vi "Dashboard Main.vi"() -> ()   [LabVIEW 2013]
uses:
  <vilib>/event_ctls.llb/eventvkey.ctl
  <vilib>/Rock Robotics/WPI/Dashboard/WPI_DashboardLogging Global.vi
  <vilib>/Utility/config.llb/Write Key (String).vi
  <vilib>/Utility/config.llb/Write Key (I32).vi
  <vilib>/Utility/config.llb/NI_LVConfig.lvlib
panel:
  out "Image Message":string="Timeout in Camera Communications"
  in  "Rec Mode":enum32{"Stop", "Record", "Playback"}(radio)
  in  "Dashboard Tab":T1(tab)
  in  "DriverValue":string(combo)
  in  "Camera Settings":T2={"Frame Rate"=30, "Compression"=30, "Size"=1} {"Frame Rate" scale=1.0..30.0; "Size" items=["640x480", "320x240", "160x120"]}
  out "MotorSliders R":cluster{"MotorSlide1":dbl, "MotorSlide2":dbl} {"MotorSlide2" scale=-1.0..1.0 scale format="%#_2e"; "MotorSlide1" scale=-1.0..1.0 scale format="%#_2e"}
  out "MotorChart R":cluster{"Numeric":dbl, "Numeric":dbl}(graph)
  out "MotorSliders L":T3 {"MotorSlide4 2" scale=0.0..14.0 scale format="%#_2e"; "MotorSlide2" scale=-1.0..1.0 scale format="%#_2e"; "MotorSlide1" scale=-1.0..1.0 scale format="%#_2e"}
  out "MotorChart L":T4(graph)
  out "JS1 Z":dbl(slide) scale=-1.0..1.0 scale format="%#_2e"
  out "Joystick 1":cluster{"X":dbl, "Y":dbl}[](graph)
  out "JS Buttons 1":T5
  out "JS2 Z":dbl(slide) scale=-1.0..1.0 scale format="%#_2e"
  out "Joystick 2":cluster{"X":dbl, "Y":dbl}[](graph)
  out "JS Buttons 2":T5
  out "Mode":T6(ring)=enum."Auto Disabled"
  out "Camera IP":string
  in  "DB Camera Config":bool
  out "fps":dbl format="%#.1g"
  out "Mbps":dbl format="%#.1g"
  out "Mbps 2":bool
  out "LED 1":bool
  in  "Slider 1":dbl(slide) scale=0.0..100.0
  in  "Checkbox 2":bool
  in  "Checkbox 1":bool
  in  "Test Slider":dbl(slide) scale=0.0..100.0 scale format="%#_3g"
  in  "On/Off":bool caption="Solenoid"
  in  "Test Name":u16(ring) items=["Select the test to run...", "Example Test", "-------------------------------", "List of tests is built in robot code.", "Replace with your own automated tests."]
  in  "Test Tree":string(tree)
  in  "Motor":cluster{"Value":dbl, "Enable":bool} {"Value" scale=-1.0..1.0 scale format="%#_3g"}
  out "Progress":T7 {"Test Progress" scale=0.0..100.0}
  in  "Rev/Fwd":cluster{"Forward":bool, "Reverse":bool}
  in  "Test Ring":u16(ring) items=["Auto", "Fixed indoor", "Fixed outdoor 1", "Fixed outdoor 2", "Fixed fluorescent 1", "Fixed fluorescent 2", "Hold current"]
  in  "Listbox":i32(listbox)
  out "Tree":string(tree)
  out "Camera Image":T8(plugin-control)
  in  "Enable":bool
  # "Left"
  # "Front"
  # "Right"
  # "Battery"
  # "Customize by placing controls and indicators here and name to\nmatch Dashboard Variables on robot."
  # "This tab is a great place for autonomous settings and validation.\nCustomize by placing controls and indicators here and name to\nmatch Dashboard Variables on robot."
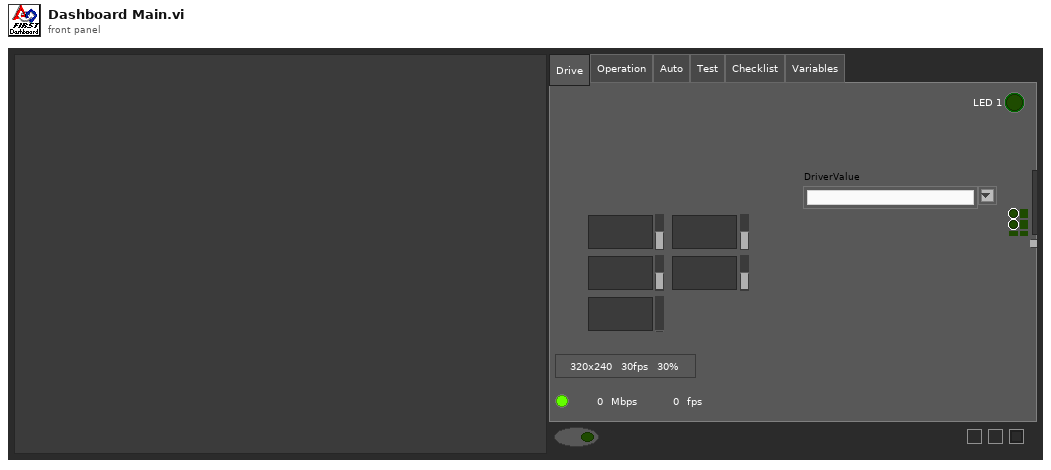
[diagram p1: front panel]
types:
  T1 = enum32{"Drive", "Operation", "Auto", "Test", "Checklist", "Variables"}
  T2 = cluster{"Frame Rate":i32, "Compression":i32, "Size":u16}
  T3 = cluster{"MotorSlide1":dbl, "MotorSlide2":dbl, "MotorSlide4 2":dbl}
  T4 = cluster{"Numeric":dbl, "Numeric":dbl, "Battery":sgl}
  T5 = cluster{bool, bool, bool, bool, bool, bool, bool, bool, bool, bool, bool, bool}
  T6 = enum8{"Tele-Op Disabled", "Tele-Op Enabled", "Auto Disabled", "Auto Enabled", "Test Disabled", "Test Enabled", ""}
  T7 = cluster{"Test Progress":u8, "Test Progress Text":string}
  T8 = typedef "IMAQ Image.ctl" = refnum<image>
  T9 = typedef "Image Type" = u32
  T10 = cluster{"Digital Inputs":bool[], "Digital Outputs":bool[]}
  T11 = cluster{"Competition mode":bool, "Robot Link":bool, "Autonomous":bool, "Enabled":bool, "E-Stop":bool, "Simulated":bool, "TestMode":bool, "Docked Window":bool}
  T12 = cluster{"Boolean Array[0]":bool, "Boolean Array[1]":bool, "Boolean Array[2]":bool, "Boolean Array[3]":bool, "Boolean Array[4]":bool, "Boolean Array[5]":bool, "Boolean Array[6]":bool, "Boolean Array[7]":bool, "Boolean Array[8]":bool, "Boolean Array[9]":bool, "Boolean Array[10]":bool, "Boolean Array[11]":bool}
  T13 = typedef "NI_LVConfig.lvlib/Config Data RefNum.ctl" = refnum<k1>
  T14 = typedef "eventvkey.ctl" = enum16{"ASCII", "Enter", "Return", "Shift", "Ctrl", "Alt", "Cmd", "Opt", "Caps", "NumLock", "Clear", "Break", "Up", "Down", "Left", "Right", "Insert", "Delete", "Home", "End", "PageUp", "PageDown", "Escape", "Help", "Pause", "ScrollLock", "F1", "F2", "F3", "F4", "F5", "F6", "F7", "F8", "F9", "F10", "F11", "F12", "F13", "F14", "F15", "F16", "F17", "F18", "F19", "F20", "F21", "F22", "F23", "F24", "Play", "VolumeUp", "VolumeDown", "Mute", "Two Byte Char"}
  T15 = cluster{"Image Size":bool, "Image Type":bool, "Pixel Value":bool, "ROI Information":bool, "Zoom Factor":bool}
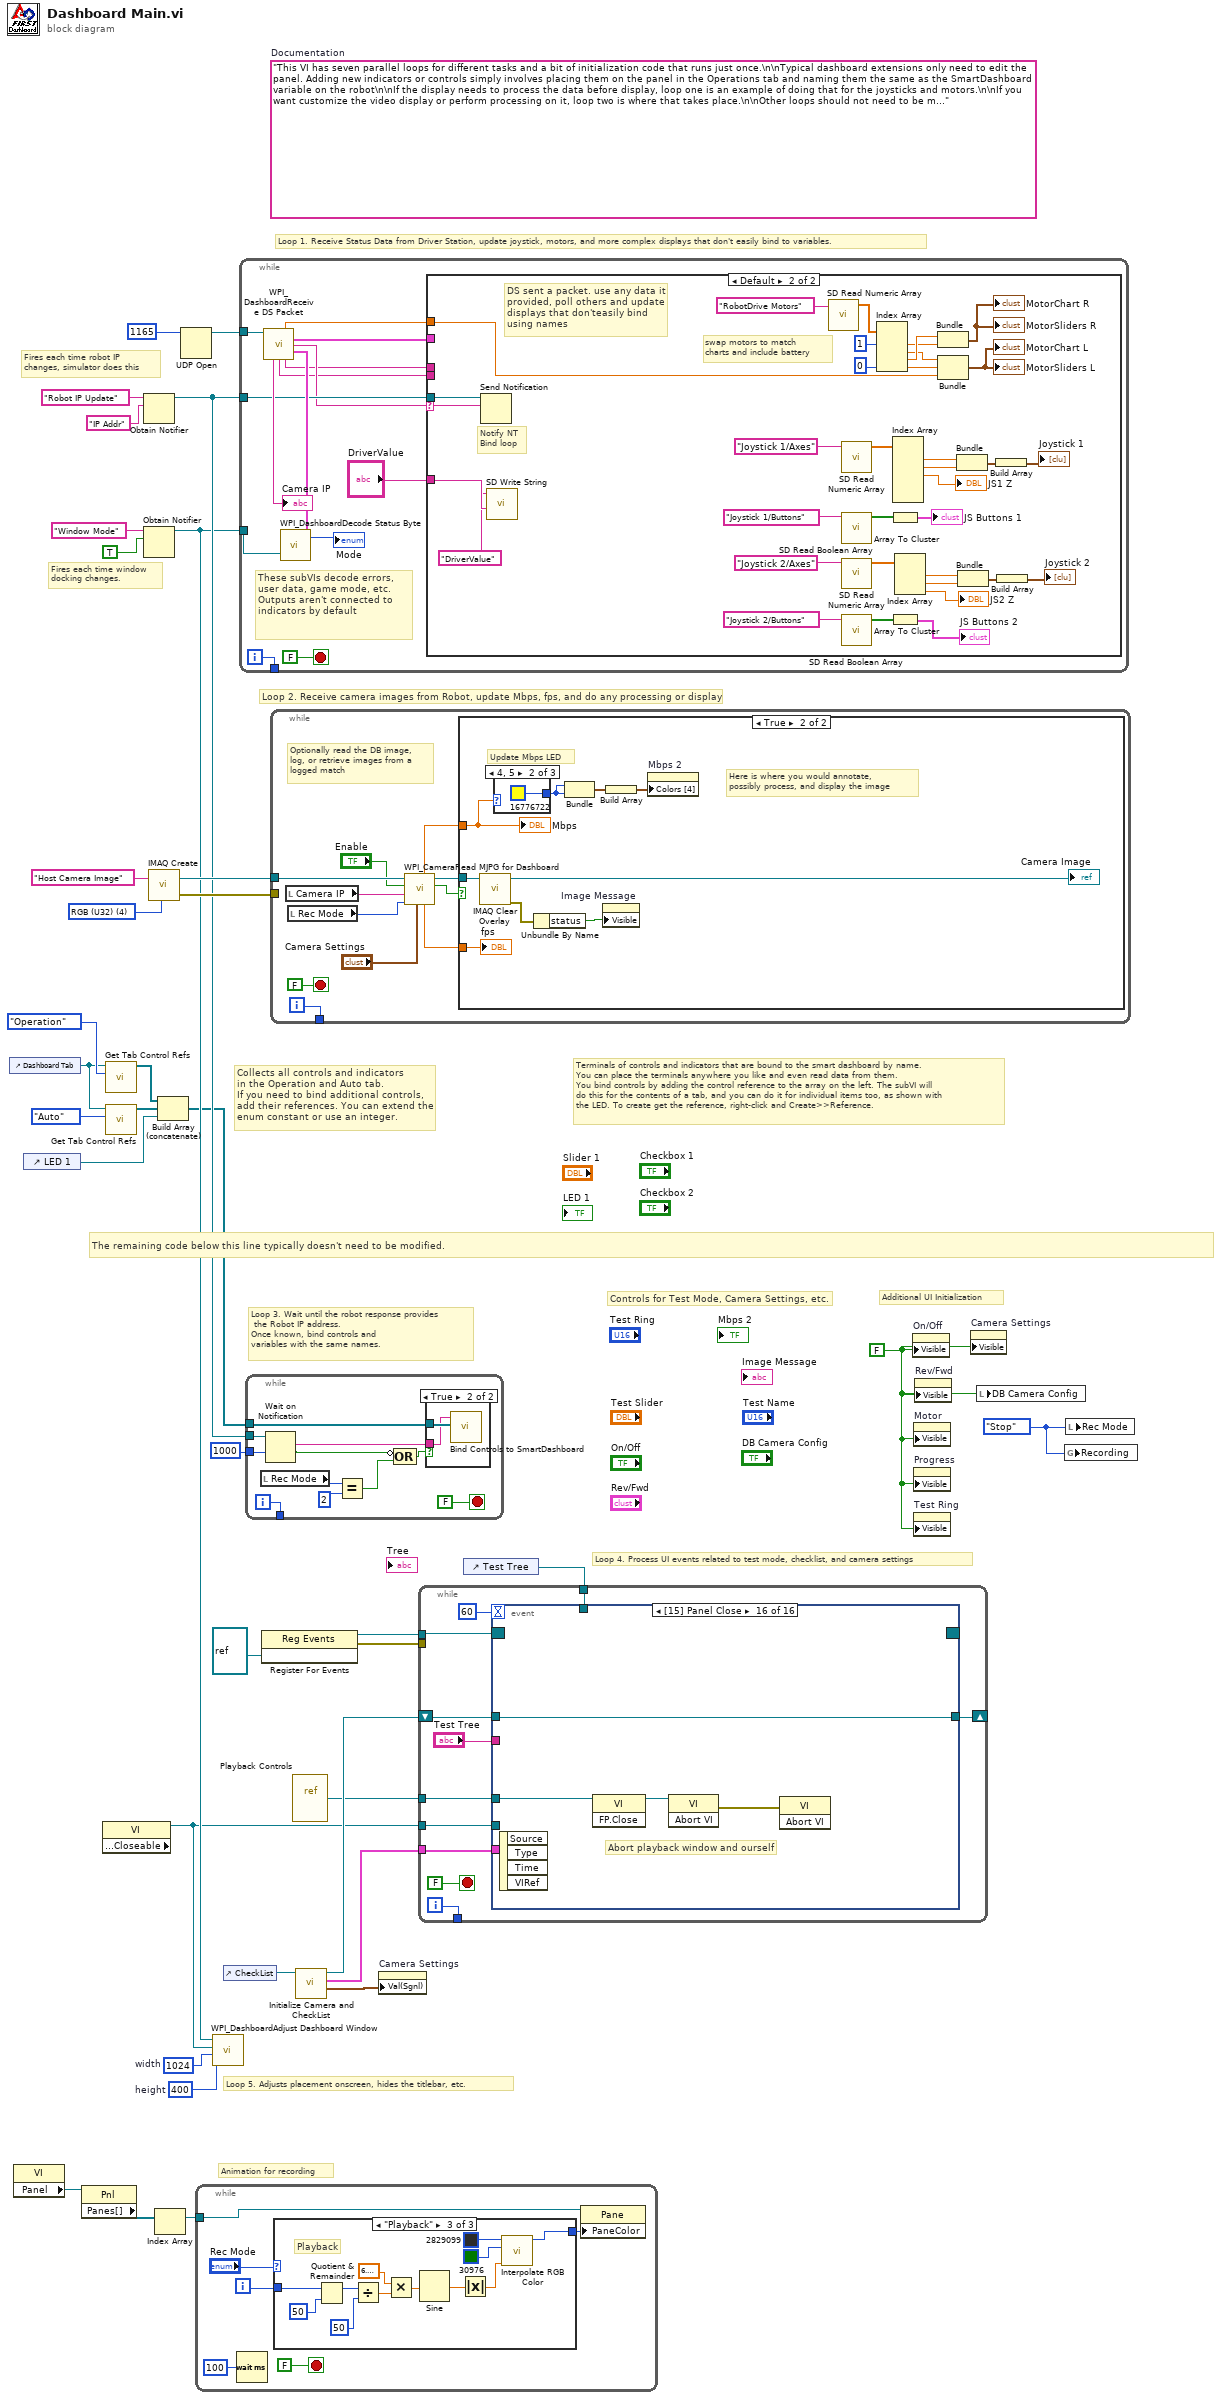
[diagram p0: block diagram]
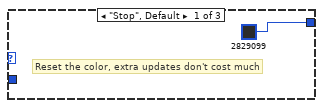
[diagram p2: hidden frame]
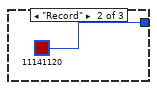
[diagram p3: hidden frame]
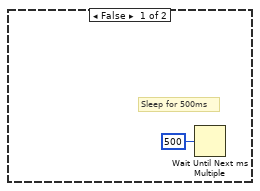
[diagram p5: hidden frame]
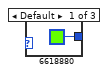
[diagram p6: hidden frame]
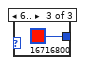
[diagram p7: hidden frame]
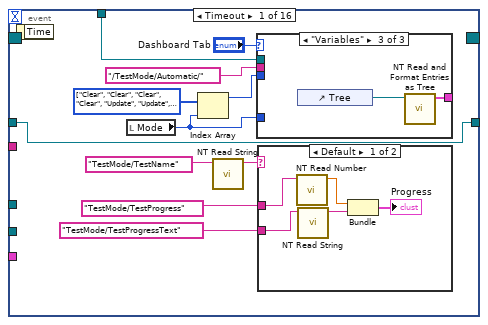
[diagram p8: hidden frame]
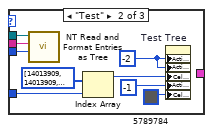
[diagram p10: hidden frame]
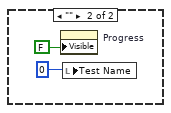
[diagram p11: hidden frame]
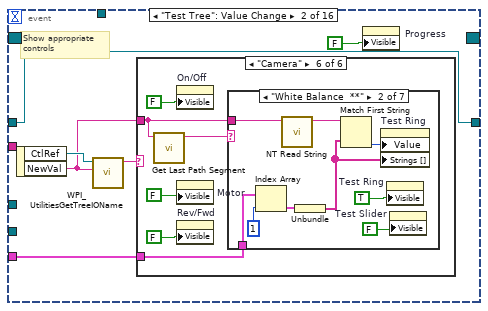
[diagram p12: hidden frame]
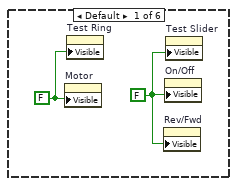
[diagram p13: hidden frame]
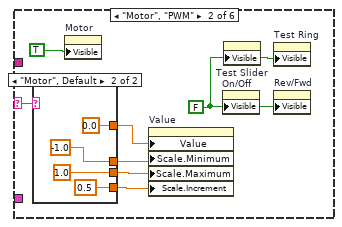
[diagram p14: hidden frame]
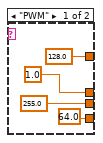
[diagram p15: hidden frame]
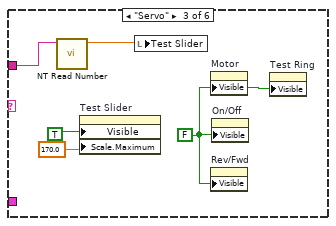
[diagram p16: hidden frame]
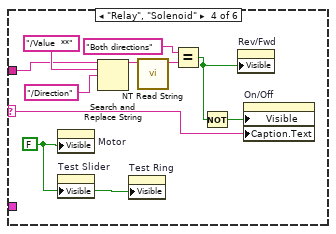
[diagram p17: hidden frame]
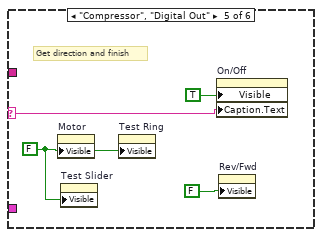
[diagram p18: hidden frame]
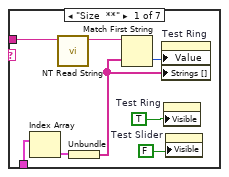
[diagram p19: hidden frame]
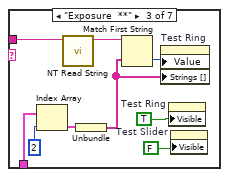
[diagram p20: hidden frame]
diagram:
  w8 = enum32{"Stop", "Record", "Playback"}."Stop" ("Rec Mode")
  w11 = 400  # height
  w12 = 1024  # width
  w25 = FALSE ("Visible")
  (unwired) "This VI has seven parallel loops for different tasks and a bit of initialization code that runs just once.\n\nTypical dashboard extensions only need to edit the panel. Adding new indicators or controls simply involves placing them on the panel in the Operations tab and naming them the same as the SmartDashboard variable on the robot\n\nIf the display needs to process the data before display, loop one is an example of doing that for the joysticks and motors.\n\nIf you want customize the video display or perform processing on it, loop two is where that takes place.\n\nOther loops should not need to be modified. They are pretty standard, and document the task they perform."  # Documentation
  w35 = T9 4 items=["Grayscale (U8)", "Grayscale (I16)", "Grayscale (SGL)", "Complex (CSG)", "RGB (U32)", "HSL (U32)", "RGB (U64)"] ("Image Type")
  # "Controls for Test Mode, Camera Settings, etc."
  # "Additional UI Initialization"
  # "Animation for recording"
  # "Fires each time robot IP\nchanges, simulator does this"
  # "Fires each time window\ndocking changes."
  # "Collects all controls and indicators\nin the Operation and Auto tab.\nIf you need to bind additional controls,\nadd their references. You can extend the\nenum constant or use an integer."
  # "The remaining code below this line typically doesn't need to be modified."
  # "Loop 4. Process UI events related to test mode, checklist, and camera settings"
  # "Terminals of controls and indicators that are bound to the smart dashboard by name.\nYou can place the terminals anywhere you like and even read data from them.\nYou bind controls by adding the control reference to the array on the left. The subVI will\ndo this for the contents of a tab, and you can do it for individual items too, as shown with\nthe LED. To create get the reference, right-click and Create>>Reference."
  # "Loop 3. Wait until the robot response provides\n the Robot IP address.\nOnce known, bind controls and\nvariables with the same names."
  # "Loop 5. Adjusts placement onscreen, hides the titlebar, etc."
  # "Loop 1. Receive Status Data from Driver Station, update joystick, motors, and more complex displays that don't easily bind to variables."
  # "Loop 2. Receive camera images from Robot, update Mbps, fps, and do any processing or display"
  n1 = control-ref of="Dashboard Tab"() -> (w6:refnum<vi>)
  n2 = property class="VI"() -> ("Panel"=w19:refnum<vi>)  [unwired: 2 in, 2 out]
  n3 = control-ref of="LED 1"() -> (w1:refnum<vi>)
  n4 = property class="Pnl"(reference=w19) -> ("Panes[]"=w20:refnum<vi>[])  [unwired: 1 in, 2 out]
  n5 = property class="VI" props=["Front Panel.Closeable"]() -> (reference out=w7:refnum<vi>)  [unwired: 2 in, 2 out]
  n6 = call <vilib>:"Get Tab Control Refs.vi"("Page Index"=T1."Operation" ("Dashboard Tab"), "TabControl in"=w6) -> ("ControlsOnPage"=w4:refnum<vi>[])  [unwired: 9 in]
  n7 = call <vilib>:"Get Tab Control Refs.vi"("Page Index"=T1."Auto" ("Dashboard Tab"), "TabControl in"=w6) -> ("ControlsOnPage"=w5:refnum<vi>[])  [unwired: 9 in]
  n8 = Obtain Notifier(name (unnamed)="Robot IP Update", notification data type="IP Addr" ("name (unnamed)")) -> (notifier out=w29:refnum<notifier>)  [unwired: 2 in, 2 out]
  n9 = Obtain Notifier(name (unnamed)="Window Mode", notification data type=TRUE) -> (notifier out=w10:refnum<notifier>)  [unwired: 2 in, 2 out]
  n10 = call "IMAQ Create"("Image Name"="Host Camera Image", "Image Type"=w35) -> ("New Image"=w33:T8, "error out"=w32:errorcluster)  [unwired: 2 in, 1 out]
  n11 = Index Array(array=w20) -> (element=w18:refnum<vi>)  [unwired: 1 in]
  n12 = Build Array (concatenate)(w4, w5, w1) -> (w3:refnum<vi>[])
  n13 = UDP Open(11:u16 1165 ("port")) -> (port=w36:refnum<k16>)  [unwired: 2 in, 4 out]
  n14 = while {
    tunnel: w18 -> [w39]
    i -> [w42]
    stop <- FALSE stop-if-true
    n15 = Wait (ms)(milliseconds to wait=u32 100) -> ()  [unwired: 1 out]
    n16 = case shown="\"Playback\"" "Rec Mode" {
      tunnel: w42 -> [_ _ w57]
      tunnel: [u32 2829099 ("Base Color") u32 11141120 ("Target Color") w46] -> w38
      frame "Stop", Default {
        # "Reset the color, extra updates don't cost much"
      }
      frame "Record" {
      }
      frame "Playback" {
        # "Playback"
        n17 = Quotient & Remainder(x=w57, y=u32 50 ("milliseconds to wait")) -> (x-y*floor(x/y)=w53:u32)  [unwired: 1 out]
        n18 = Divide(x=w53, y=u32 50 ("milliseconds to wait")) -> (x/y=w50:dbl)
        n19 = Multiply(x=6.283185307179586, y=w50) -> (x*y=w55:dbl)
        n20 = Sine(x=w55) -> (sin(x)=w54:dbl)
        n21 = Absolute Value(x=w54) -> (abs(x)=w47:dbl)
        n22 = call "Interpolate RGB Color.vi"("Proportion"=w47, "Target Color"=u32 30976, "Base Color"=u32 2829099) -> ("Result Color"=w46:u32)  [unwired: 8 in]
      }
    }
    n23 = property class="Pane"(reference=w39, "PaneColor"=w38) -> ()  [unwired: 1 in, 2 out]
  }
  n24 = call <vilib>:"WPI_DashboardAdjust Dashboard Window.vi"("height"=w11, "width"=w12, "reference in"=w7, "Notifier in"=w10) -> ()  [unwired: 8 in]
  n25 = control-ref of="CheckList"() -> (w9:refnum<vi>)
  n26 = while {
    tunnel: w36 -> [w69]
    tunnel: w29 -> [w64]
    tunnel: w10 -> [w68]
    tunnel: [w65] -> _
    i -> [w65]
    stop <- FALSE stop-if-true
    # "These subVIs decode errors, user data, game mode, etc.\nOutputs aren't connected to indicators by default"
    n27 = call <vilib>:"WPI_DashboardReceive DS Packet.vi"("Recv Socket"=w69) -> ("Battery"=w59:sgl, "Driver Station"=w60:T10, "Robot IP Address"=w63:string, "Status"=w70:T11, "Camera IP Address"=→"Camera IP":string, "Low Priority User Data"=w62:string, "High Priority User Data"=w61:string)  [unwired: 1 in, 7 out]
    n28 = call <vilib>:"WPI_DashboardDecode Status Byte.vi"("Window Mode Notifier"=w68, "Status"=w70) -> ("Mode"=→"Mode":T6)  [unwired: 1 out]
    n29 = case shown="Default" w63 {
      selector: w63 -> [_ w84]
      tunnel: w64 -> [_ w85]
      tunnel: w62 -> [_ _]
      tunnel: w61 -> [_ _]
      tunnel: w60 -> [_ _]
      tunnel: w59 -> [_ w83]
      tunnel: "DriverValue" -> [_ w73]
      frame "0.0.0.0" {
        # "DS not sending packets, or no robot exists yet.\nDon't poll the variables"
      }
      frame Default {
        # "Notify NT\nBind loop"
        # "DS sent a packet. use any data it\nprovided, poll others and update\ndisplays that don'teasily bind\nusing names"
        # "swap motors to match\ncharts and include battery"
        n30 = Send Notification(notification=w84, notifier=w85) -> ()  [unwired: 1 in, 2 out]
        n31 = call <vilib>:"SD Write String.vi"("String"=w73, "Name"="DriverValue") -> ()  [unwired: 8 in, 2 out]
        n32 = call <vilib>:"SD Read Numeric Array.vi"("Name"="RobotDrive Motors") -> ("Numeric Array"=w82:dbl[])  [unwired: 8 in, 2 out]
        n33 = call <vilib>:"SD Read Numeric Array.vi"("Name"="Joystick 1/Axes") -> ("Numeric Array"=w101:dbl[])  [unwired: 8 in, 2 out]
        n34 = call <vilib>:"SD Read Boolean Array.vi"("Name"="Joystick 1/Buttons") -> ("Boolean Array"=w103:bool[])  [unwired: 8 in, 2 out]
        n35 = call <vilib>:"SD Read Numeric Array.vi"("Name"="Joystick 2/Axes") -> ("Numeric Array"=w95:dbl[])  [unwired: 8 in, 2 out]
        n36 = call <vilib>:"SD Read Boolean Array.vi"("Name"="Joystick 2/Buttons") -> ("Boolean Array"=w94:bool[])  [unwired: 8 in, 2 out]
        n37 = Index Array(array=w82, index #1=1, index #4=0) -> (element #1=w78:dbl, element #2=w77:dbl, element #3=w79:dbl, element #4=w74:dbl)  [unwired: 2 in]
        n38 = Array To Cluster(array=w103) -> (cluster=→"JS Buttons 1":T12)
        n39 = Array To Cluster(array=w94) -> (cluster=→"JS Buttons 2":T12)
        n40 = Index Array(array=w101) -> (element #1=w98:dbl, element #2=w99:dbl, element #3=→"JS1 Z":dbl)  [unwired: 6 in, 3 out]
        n41 = Index Array(array=w95) -> (element #1=w90:dbl, element #2=w89:dbl, element #3=→"JS2 Z":dbl)  [unwired: 3 in]
        n42 = Bundle("Numeric"=w79, "Numeric"=w78) -> (→"MotorChart R" →"MotorSliders R":cluster{"Numeric":dbl, "Numeric":dbl})  [unwired: 1 in]
        n43 = Bundle("Numeric"=w77, "Numeric"=w74, "Battery"=w83) -> (→"MotorChart L" →"MotorSliders L":T4)  [unwired: 1 in]
        n44 = Bundle("Numeric"=w98, "Numeric"=w99) -> (w97:cluster{"Numeric":dbl, "Numeric":dbl})  [unwired: 1 in]
        n45 = Bundle("Numeric"=w90, "Numeric"=w89) -> (w91:cluster{"Numeric":dbl, "Numeric":dbl})  [unwired: 1 in]
        n46 = Build Array(w97) -> (→"Joystick 1":cluster{"Numeric":dbl, "Numeric":dbl}[])
        n47 = Build Array(w91) -> (→"Joystick 2":cluster{"Numeric":dbl, "Numeric":dbl}[])
      }
    }
  }
  n48 = while {
    tunnel: w3 -> [w117]
    tunnel: w29 -> [w115]
    tunnel: [w113] -> _
    tunnel: u32 1000 ("milliseconds to wait") -> [w112]
    i -> [w113]
    stop <- FALSE stop-if-true
    n49 = local read "Rec Mode"() -> (w108:enum32{"Stop", "Record", "Playback"})
    n50 = Wait on Notification(notifier=w115, timeout in ms (-1)=w112) -> (notification=w114:string, timed out?=w110:bool)  [unwired: 2 in, 2 out]
    n51 = Equal?(x=w108, y=u16 2 ("Rec Mode")) -> (x = y?=w109:bool)
    n52 = Compound Arithmetic op=OR(invert w110, w109) -> (w111:bool)
    n53 = case shown="True" w111 {
      tunnel: w117 -> [_ w119]
      tunnel: w114 -> [_ w118]
      frame False {
      }
      frame True {
        n54 = call <vilib>:"Bind Controls to SmartDashboard.vi"("Bound Control Refs"=w119, "Server IP Address"=w118) -> ()  [unwired: 10 in]
      }
    }
  }
  n55 = register-events(refnum<vi> refnum) -> (reference out=w16:refnum<event-registration>, error out=w15:errorcluster)  [unwired: 2 in]
  n56 = while {
    tunnel: w33 -> [w128]
    tunnel: w32 -> [_]
    tunnel: [w129] -> _
    i -> [w129]
    stop <- FALSE stop-if-true
    # "Optionally read the DB image,\nlog, or retrieve images from a\nlogged match"
    n57 = local read "Camera IP"() -> (w121:string)
    n58 = local read "Rec Mode"() -> (w120:enum32{"Stop", "Record", "Playback"})
    n59 = call <vilib>:"WPI_CameraRead MJPG for Dashboard.vi"("Camera Settings"="Camera Settings", "Rec Mode"=w120, "Camera IP"=w121, "Enable"="Enable", "Refnum in"=w128) -> ("Active"=w125:bool, "Refnum out"=w127:T8, "FPS"=w124:dbl, "Bandwidth (Mbps)"=w123:dbl)  [unwired: 3 in]
    n60 = case shown="True" w125 {
      tunnel: w127 -> [_ w135]
      tunnel: w123 -> [_ w134]
      tunnel: w124 -> [_ w132]
      frame False {
        # "Sleep for 500ms"
        n61 = Wait Until Next ms Multiple(millisecond multiple=u32 500) -> ()  [unwired: 1 out]
      }
      frame True {
        # "Here is where you would annotate,\npossibly process, and display the image"
        # "Update Mbps LED"
        n62 = call "IMAQ Clear Overlay"("Image"=w135) -> ("error out"=w139:errorcluster, "Image Out"=→"Camera Image":T8)  [unwired: 2 in, 7 out]
        n63 = case shown="4, 5" w134 {
          tunnel: [u32 6618880 ("Color Box") u32 16776722 ("Color Box") u32 16716800 ("Color Box")] -> w136
          frame Default {
          }
          frame 4, 5 {
          }
          frame 6.. {
          }
        }
        n64 = Unbundle By Name(w139) -> ("status"=w140:bool)
        n65 = Bundle("Color Box"=w136, "Color Box"=w136) -> (w138:cluster{"Color Box":u32, "Color Box":u32})  [unwired: 1 out]
        n66 = property on="Image Message" class="Str"("Visible"=w140) -> ()  [unwired: 2 in, 2 out]
        n67 = Build Array(w138) -> (w137:cluster{"Color Box":u32, "Color Box":u32}[])
        n68 = property on="Mbps 2" class="Bool (strict)"("Colors [4]"=w137) -> ()  [unwired: 2 in, 2 out]
        "Mbps" <- w134
        "fps" <- w132
      }
    }
  }
  n69 = vi-ref "Playback Controls.vi"() -> (w17:refnum<vi>)
  n70 = call "Initialize Camera and CheckList.vi"("ListBox in"=w9) -> ("Cluster"=w23:cluster{"value":i32, "value":i32, "index":i32}, "Array"=w24:cluster{string[]}[], "File Refnum"=w22:T13)  [unwired: 8 in]
  n71 = property on="Camera Settings" class="Clust (strict)"("Val(Sgnl)"=w23) -> ()  [unwired: 2 in, 2 out]
  n72 = control-ref of="Test Tree"() -> (w21:refnum<vi>)
  n73 = while {
    tunnel: w24 -> [w151]
    shift-right: [w150] -> _
    shift-left: w22 -> [w149]
    tunnel: [w148] -> _
    tunnel: w21 -> [w147]
    tunnel: w17 -> [w146]
    tunnel: w16 -> [w145]
    tunnel: w15 -> [_]
    tunnel: w7 -> [w144]
    i -> [w148]
    stop <- FALSE stop-if-true
    n74 = event shown="[15] Panel Close" {
      selector: w145 -> [_ _ _ _ _ _ _ _ _ _ _ _ _ _ _ _]
      dyn-events: [_ _ _ _ _ _ _ _ _ _ _ _ _ w389 _ _] -> _
      timeout: u32 60 ("milliseconds to wait") -> [_ _ _ _ _ _ _ _ _ _ _ _ _ _ _ _]
      tunnel: w147 -> [w161 _ _ _ _ _ _ _ _ _ _ _ _ _ _ _]
      tunnel: "Test Tree" -> [_ _ _ _ _ _ _ _ w358 w366 w368 w372 w380 _ _ _]
      tunnel: w151 -> [_ w185 _ _ _ _ w322 w352 _ _ _ _ _ _ _ _]
      tunnel: [w155 w184 w283 w288 w296 w308 w321 w345 w357 w364 w367 w371 w379 w391 w405 w406] -> w150
      tunnel: w149 -> [w155 w184 w283 w288 w296 w308 w320 w345 w357 w364 w367 w371 w379 w391 w405 w406]
      tunnel: w146 -> [_ _ _ _ _ _ _ _ _ _ _ _ _ w392 _ w409]
      tunnel: w144 -> [_ _ _ _ _ _ _ _ _ _ _ _ _ w387 _ _]
      event Timeout {
        w160 = enum16{"Update", "Clear"}[] [enum."Clear", enum."Clear", enum."Clear", enum."Clear", enum."Update", enum."Update", enum."Clear"] items=["Update", "Clear"]
        n75 = event-data() -> ()  [unwired: 1 in, 1 out]
        n76 = local read "Mode"() -> (w158:T6)
        n77 = Index Array(array=w160, index=w158) -> (element=w159:enum16{"Update", "Clear"})
        n78 = call <vilib>:"NT Read String.vi"("Name"="TestMode/TestName") -> ("String"=w164:string)  [unwired: 9 in, 1 out]
        n79 = case shown="\"Variables\"" "Dashboard Tab" {
          tunnel: w161 -> [_ w174 _]
          tunnel: "/TestMode/Automatic/" ("Name Pattern") -> [_ w173 _]
          tunnel: w159 -> [_ w172 _]
          tunnel: w158 -> [_ w170 _]
          tunnel: [_ _ w176] -> _
          frame "Operation", Default {
          }
          frame "Test" {
            w169 = -2 ("Active Item:Row Number")
            n80 = call <vilib>:"NT Read and Format Entries as Tree.vi"("Operation"=w172, "Name Pattern"=w173, "Tree Refnum"=w174) -> ()  [unwired: 7 in, 2 out]
            n81 = Index Array(array=u32[] [14013909, 14013909, 14013909, 14013909, 14013909, 16777215, 14013909], index=w170) -> (element=w168:u32)
            n82 = property on="Test Tree" class="Tree (strict)"("Active Item Row Number"=w169, "ActiveColNum"=w169, "CellBG"=w168, "Active Item Row Number"=-1 ("Active Item:Row Number"), "CellBG"=u32 5789784 ("Color Box")) -> ()  [unwired: 2 in, 2 out]
          }
          frame "Variables" {
            n83 = control-ref of="Tree"() -> (w175:refnum<vi>)
            n84 = call <vilib>:"NT Read and Format Entries as Tree.vi"("Tree Refnum"=w175) -> ("Formatted Strings"=w176:cluster{"Name":string, "Value":string}[])  [unwired: 9 in, 1 out]
          }
        }
        n85 = case shown="Default" w164 {
          tunnel: "TestMode/TestProgress" ("Name") -> [w178 _]
          tunnel: "TestMode/TestProgressText" ("Name") -> [w177 _]
          frame Default {
            n86 = call <vilib>:"NT Read Number.vi"("Name"=w178) -> ("Numeric"=w179:dbl)  [unwired: 9 in, 1 out]
            n87 = call <vilib>:"NT Read String.vi"("Name"=w177) -> ("String"=w180:string)  [unwired: 9 in, 1 out]
            n88 = Bundle("Numeric"=w179, "String"=w180) -> (→"Progress":cluster{"Numeric":dbl, "String":string})  [unwired: 1 in]
          }
          frame "" {
            n89 = property on="Progress" class="Clust (strict)"("Visible"=FALSE) -> ()  [unwired: 2 in, 2 out]
            n90 = local write "Test Name"(u16 0) -> ()
          }
        }
      }
      event "Test Tree": Value Change {
        # "Show appropriate\ncontrols"
        n91 = event-data() -> ("CtlRef"=w188:refnum<vi>, "NewVal"=w186:string)  [unwired: 1 in]
        n92 = call <vilib>:"WPI_UtilitiesGetTreeIOName.vi"("NewVal"=w186, "TreeControl in"=w188) -> ("I/O Name"=w189:string)  [unwired: 9 in]
        n93 = case shown="\"Camera\"" w189 {
          selector: w189 -> [_ w196 _ w214 w223 _]
          tunnel: w186 -> [_ _ w211 w213 _ w230]
          tunnel: w185 -> [_ _ _ _ _ w229]
          frame Default {
            w191 = FALSE ("Visible")
            w190 = FALSE ("Visible")
            n94 = property on="Motor" class="Clust (strict)"("Visible"=w190) -> ()  [unwired: 2 in, 2 out]
            n95 = property on="Test Ring" class="Ring (strict)"("Visible"=w190) -> ()  [unwired: 2 in, 2 out]
            n96 = property on="Rev/Fwd" class="Clust (strict)"("Visible"=w191) -> ()  [unwired: 2 in, 2 out]
            n97 = property on="On/Off" class="Bool (strict)"("Visible"=w191) -> ()  [unwired: 2 in, 2 out]
            n98 = property on="Test Slider" class="Slide (strict)"("Visible"=w191) -> ()  [unwired: 2 in, 2 out]
          }
          frame "Motor", "PWM" {
            w197 = FALSE ("Visible")
            n99 = case shown="\"Motor\", Default" w196 {
              tunnel: [1.0 ("Value") -1.0 ("Value")] -> w195
              tunnel: [255.0 ("Value") 1.0 ("Value")] -> w194
              tunnel: [128.0 ("Value") 0.0 ("Value")] -> w193
              tunnel: [64.0 ("Value") 0.5 ("Value")] -> w192
              frame "PWM" {
              }
              frame "Motor", Default {
              }
            }
            n100 = property on="Motor" class="Clust (strict)"("Visible"=TRUE) -> ()  [unwired: 2 in, 2 out]
            n101 = property on="Value" class="Slide (strict)"("Value"=w193, "Scale.Minimum"=w195, "Scale.Maximum"=w194, "Scale.Increment"=w192) -> ()  [unwired: 2 in, 2 out]
            n102 = property on="On/Off" class="Bool (strict)"("Visible"=w197) -> ()  [unwired: 2 in, 2 out]
            n103 = property on="Test Slider" class="Slide (strict)"("Visible"=w197) -> ()  [unwired: 2 in, 2 out]
            n104 = property on="Test Ring" class="Ring (strict)"("Visible"=w197) -> ()  [unwired: 2 in, 2 out]
            n105 = property on="Rev/Fwd" class="Clust (strict)"("Visible"=w197) -> ()  [unwired: 2 in, 2 out]
          }
          frame "Servo" {
            w209 = FALSE ("Visible")
            n106 = call <vilib>:"NT Read Number.vi"("Name"=w211) -> ("Numeric"=w210:dbl)  [unwired: 9 in, 1 out]
            n107 = property on="Test Slider" class="Slide (strict)"("Visible"=TRUE, "Scale.Maximum"=170.0 ("Scale.Range:Maximum")) -> ()  [unwired: 2 in, 2 out]
            n108 = local write "Test Slider"(w210) -> ()
            n109 = property on="Motor" class="Clust (strict)"("Visible"=w209) -> ()  [unwired: 2 in, 2 out]
            n110 = property on="Rev/Fwd" class="Clust (strict)"("Visible"=w209) -> ()  [unwired: 2 in, 2 out]
            n111 = property on="On/Off" class="Bool (strict)"("Visible"=w209) -> ()  [unwired: 2 in, 2 out]
            n112 = property on="Test Ring" class="Ring (strict)"("Visible"=w209) -> ()  [unwired: 2 in, 2 out]
          }
          frame "Relay", "Solenoid" {
            w212 = FALSE ("Visible")
            n113 = property on="Motor" class="Clust (strict)"("Visible"=w212) -> ()  [unwired: 2 in, 2 out]
            n114 = property on="Test Slider" class="Slide (strict)"("Visible"=w212) -> ()  [unwired: 2 in, 2 out]
            n115 = Search and Replace String(input string=w213, search string="/Value  **", replace string="/Direction") -> (result string=w219:string)  [unwired: 5 in, 3 out]
            n116 = property on="Test Ring" class="Ring (strict)"("Visible"=w212) -> ()  [unwired: 2 in, 2 out]
            n117 = call <vilib>:"NT Read String.vi"("Name"=w219) -> ("String"=w217:string)  [unwired: 9 in, 1 out]
            n118 = Equal?(x="Both directions", y=w217) -> (x = y?=w215:bool)
            n119 = Not(x=w215) -> (.not. x?=w216:bool)
            n120 = property on="Rev/Fwd" class="Clust (strict)"("Visible"=w215) -> ()  [unwired: 2 in, 2 out]
            n121 = property on="On/Off" class="Bool (strict)"("Visible"=w216, "Caption.Text"=w214) -> ()  [unwired: 2 in, 2 out]
          }
          frame "Compressor", "Digital Out" {
            w222 = FALSE ("Visible")
            # "Get direction and finish"
            n122 = property on="Motor" class="Clust (strict)"("Visible"=w222) -> ()  [unwired: 2 in, 2 out]
            n123 = property on="Test Slider" class="Slide (strict)"("Visible"=w222) -> ()  [unwired: 2 in, 2 out]
            n124 = property on="Test Ring" class="Ring (strict)"("Visible"=w222) -> ()  [unwired: 2 in, 2 out]
            n125 = property on="On/Off" class="Bool (strict)"("Visible"=TRUE, "Caption.Text"=w223) -> ()  [unwired: 2 in, 2 out]
            n126 = property on="Rev/Fwd" class="Clust (strict)"("Visible"=FALSE) -> ()  [unwired: 2 in, 2 out]
          }
          frame "Camera" {
            n127 = call <vilib>:"Get Last Path Segment.vi"("String in"=w230) -> ("String out"=w231:string)  [unwired: 10 in]
            n128 = property on="On/Off" class="Bool (strict)"("Visible"=FALSE) -> ()  [unwired: 2 in, 2 out]
            n129 = property on="Motor" class="Clust (strict)"("Visible"=FALSE) -> ()  [unwired: 2 in, 2 out]
            n130 = property on="Rev/Fwd" class="Clust (strict)"("Visible"=FALSE) -> ()  [unwired: 2 in, 2 out]
            n131 = case shown="\"White Balance  **\"" w231 {
              tunnel: w230 -> [w237 w246 w255 w264 w273 _ w279]
              tunnel: w229 -> [w235 w243 w252 w261 w270 _ _]
              frame "Size  **" {
                n132 = Index Array(array=w235) -> (element=w234:cluster{string[]})  [unwired: 1 in]
                n133 = call <vilib>:"NT Read String.vi"("Name"=w237) -> ("String"=w236:string)  [unwired: 9 in, 1 out]
                n134 = Unbundle(w234) -> (w232:string[])
                n135 = Match First String(2:w232, 3:w236) -> (0:w233:i32)  [unwired: 1 out]
                n136 = property on="Test Ring" class="Ring (strict)"("Value"=w233, "Strings []"=w232) -> ()  [unwired: 2 in, 2 out]
                n137 = property on="Test Ring" class="Ring (strict)"("Visible"=TRUE) -> ()  [unwired: 2 in, 2 out]
                n138 = property on="Test Slider" class="Slide (strict)"("Visible"=FALSE) -> ()  [unwired: 2 in, 2 out]
              }
              frame "White Balance  **" {
                n139 = Index Array(array=w243, index=1) -> (element=w244:cluster{string[]})
                n140 = call <vilib>:"NT Read String.vi"("Name"=w246) -> ("String"=w245:string)  [unwired: 9 in, 1 out]
                n141 = Unbundle(w244) -> (w241:string[])
                n142 = Match First String(2:w241, 3:w245) -> (0:w240:i32)  [unwired: 1 out]
                n143 = property on="Test Ring" class="Ring (strict)"("Value"=w240, "Strings []"=w241) -> ()  [unwired: 2 in, 2 out]
                n144 = property on="Test Ring" class="Ring (strict)"("Visible"=TRUE) -> ()  [unwired: 2 in, 2 out]
                n145 = property on="Test Slider" class="Slide (strict)"("Visible"=FALSE) -> ()  [unwired: 2 in, 2 out]
              }
              frame "Exposure  **" {
                n146 = Index Array(array=w252, index=2) -> (element=w253:cluster{string[]})
                n147 = call <vilib>:"NT Read String.vi"("Name"=w255) -> ("String"=w254:string)  [unwired: 9 in, 1 out]
                n148 = Unbundle(w253) -> (w249:string[])
                n149 = Match First String(2:w249, 3:w254) -> (0:w250:i32)  [unwired: 1 out]
                n150 = property on="Test Ring" class="Ring (strict)"("Value"=w250, "Strings []"=w249) -> ()  [unwired: 2 in, 2 out]
                n151 = property on="Test Ring" class="Ring (strict)"("Visible"=TRUE) -> ()  [unwired: 2 in, 2 out]
                n152 = property on="Test Slider" class="Slide (strict)"("Visible"=FALSE) -> ()  [unwired: 2 in, 2 out]
              }
              frame "Exposure Priority  **" {
                n153 = Index Array(array=w261, index=3) -> (element=w262:cluster{string[]})
                n154 = call <vilib>:"NT Read String.vi"("Name"=w264) -> ("String"=w263:string)  [unwired: 9 in, 1 out]
                n155 = Unbundle(w262) -> (w258:string[])
                n156 = Match First String(2:w258, 3:w263) -> (0:w259:i32)  [unwired: 1 out]
                n157 = property on="Test Ring" class="Ring (strict)"("Value"=w259, "Strings []"=w258) -> ()  [unwired: 2 in, 2 out]
                n158 = property on="Test Ring" class="Ring (strict)"("Visible"=TRUE) -> ()  [unwired: 2 in, 2 out]
                n159 = property on="Test Slider" class="Slide (strict)"("Visible"=FALSE) -> ()  [unwired: 2 in, 2 out]
              }
              frame "Color Enable  **" {
                n160 = Index Array(array=w270, index=4) -> (element=w271:cluster{string[]})
                n161 = call <vilib>:"NT Read String.vi"("Name"=w273) -> ("String"=w272:string)  [unwired: 9 in, 1 out]
                n162 = Unbundle(w271) -> (w267:string[])
                n163 = Match First String(2:w267, 3:w272) -> (0:w268:i32)  [unwired: 1 out]
                n164 = property on="Test Ring" class="Ring (strict)"("Value"=w268, "Strings []"=w267) -> ()  [unwired: 2 in, 2 out]
                n165 = property on="Test Ring" class="Ring (strict)"("Visible"=TRUE) -> ()  [unwired: 2 in, 2 out]
                n166 = property on="Test Slider" class="Slide (strict)"("Visible"=FALSE) -> ()  [unwired: 2 in, 2 out]
              }
              frame Default {
                n167 = property on="Test Ring" class="Ring (strict)"("Visible"=FALSE) -> ()  [unwired: 2 in, 2 out]
                n168 = property on="Test Slider" class="Slide (strict)"("Visible"=FALSE) -> ()  [unwired: 2 in, 2 out]
              }
              frame "Brightness  **", "Color Level  **", "Compression  **", "FPS  **", "Sharpness  **" {
                n169 = call <vilib>:"NT Read Number.vi"("Name"=w279) -> ("Numeric"=w278:dbl)  [unwired: 9 in, 1 out]
                n170 = local write "Test Slider"(w278) -> ()
                n171 = property on="Test Ring" class="Ring (strict)"("Visible"=FALSE) -> ()  [unwired: 2 in, 2 out]
                n172 = property on="Test Slider" class="Slide (strict)"("Visible"=TRUE, "Scale.Maximum"=100.0 ("Scale.Range:Maximum")) -> ()  [unwired: 2 in, 2 out]
              }
            }
          }
        }
        n173 = property on="Progress" class="Clust (strict)"("Visible"=FALSE) -> ()  [unwired: 2 in, 2 out]
      }
      event "Test Name": Mouse Enter {
        # "Populate the ring with the list of tests"
        n174 = event-data() -> ()  [unwired: 1 in, 1 out]
        n175 = call <vilib>:"NT Read String Array.vi"("Name"="TestMode/TestList") -> ("String Array"=w287:string[])  [unwired: 9 in, 1 out]
        n176 = Build Array (concatenate)("Select the test to run...", w287) -> (w286:string[])
        n177 = property on="Test Name" class="Ring (strict)"("Strings []"=w286) -> ()  [unwired: 2 in, 2 out]
      }
      event "Test Name": Value Change {
        w289 = FALSE ("Visible")
        # "Tell the robot the test name to run"
        n178 = event-data() -> ("NewVal"=w293:u16)  [unwired: 1 in]
        n179 = property on="Test Name" class="Ring (strict)"() -> ("Strings []"=w294:string[])  [unwired: 2 in, 2 out]
        n180 = local write "Progress"(T7 {"Test Progress"=0, "Test Progress Text"=""} ("Progress")) -> ()
        n181 = Index Array(array=w294, index=w293) -> (element=w292:string)
        n182 = call <vilib>:"NT Write String.vi"("String"=w292, "Name"="TestMode/TestName") -> ()  [unwired: 9 in, 1 out]
        n183 = property on="Progress" class="Clust (strict)"("Visible"=TRUE) -> ()  [unwired: 2 in, 2 out]
        n184 = property on="Motor" class="Clust (strict)"("Visible"=w289) -> ()  [unwired: 2 in, 2 out]
        n185 = property on="Test Slider" class="Slide (strict)"("Visible"=w289) -> ()  [unwired: 2 in, 2 out]
        n186 = property on="On/Off" class="Bool (strict)"("Visible"=w289) -> ()  [unwired: 2 in, 2 out]
        n187 = property on="Rev/Fwd" class="Clust (strict)"("Visible"=w289) -> ()  [unwired: 2 in, 2 out]
        n188 = property on="Test Ring" class="Ring (strict)"("Visible"=w289) -> ()  [unwired: 2 in, 2 out]
      }
      event "Listbox": Double Click {
        n189 = event-data() -> ("PlatMods.Shift"=w297:bool, "Row"=w299:i32)  [unwired: 1 in]
        n190 = case shown="True" w297 {
          tunnel: w299 -> [w303 _]
          tunnel: 1 -> [w302 _]
          frame False {
            n191 = property on="Listbox" class="LstBox (strict)"() -> ("Item Symbols"=w301:i32[])  [unwired: 2 in, 2 out]
            n192 = Replace Array Subset(array=w301, new element=w302, index=w303) -> (w300:i32[])
            n193 = property on="Listbox" class="LstBox (strict)"("Item Symbols"=w300) -> ()  [unwired: 2 in, 2 out]
          }
          frame True {
            w304 = 0 ("Top Row")
            n194 = property on="Listbox" class="LstBox (strict)"() -> ("Number of Rows"=w306:u32)  [unwired: 2 in, 2 out]
            n195 = Initialize Array(0, w306) -> (w305:i32[])
            n196 = property on="Listbox" class="LstBox (strict)"("Top Row"=w304, "Value"=w304, "Item Symbols"=w305) -> ()  [unwired: 2 in, 2 out]
          }
        }
      }
      event "Listbox": Key Down {
        n197 = event-data() -> ("VKey"=w310:T14)  [unwired: 1 in]
        n198 = case shown="\"Left\", \"Right\"" w310 {
          selector: w310 -> [w315 _]
          tunnel: eventvkey."Left" ("VKey") -> [w313 _]
          frame "Left", "Right" {
            n199 = Equal?(x=w313, y=w315) -> (x = y?=w314:bool)
            n200 = Select(t=0, s=w314, f=1) -> (s? t:f=w316:i32)
            n201 = property on="Listbox" class="LstBox (strict)"() -> ("Item Symbols"=w319:i32[])  [unwired: 2 in, 2 out]
            n202 = Replace Array Subset(array=w319, new element=w316, index="Listbox") -> (w318:i32[])
            n203 = property on="Listbox" class="LstBox (strict)"("Item Symbols"=w318) -> ()  [unwired: 2 in, 2 out]
          }
          frame Default {
          }
        }
      }
      event "DB Camera Config": Value Change {
        n204 = event-data() -> ("NewVal"=w323:bool)  [unwired: 1 in]
        n205 = case shown="False" w323 {
          tunnel: w322 -> [w332 _]
          tunnel: [w325 w343] -> w321
          tunnel: w320 -> [w324 w343]
          frame False {
            w339 = "Camera"
            w342 = FALSE ("Visible")
            n206 = local read "Camera Settings"() -> (w331:T2)
            n207 = Index Array(array=w332) -> (element=w335:cluster{string[]})  [unwired: 1 in]
            n208 = Unbundle(w331) -> ("Frame Rate"=w330:i32, "Compression"=w329:i32, "Size"=w333:u16)
            n209 = Unbundle(w335) -> (w334:string[])
            n210 = Index Array(array=w334, index=w333) -> (element=w328:string)
            n211 = call-poly <vilib>:"Write Key.vi"("section"=w339, "value"=w328, "key"="Size", "refnum"=w324) -> ("refnum out"=w341:T13)  [unwired: 2 in, 5 out]
            n212 = call-poly <vilib>:"Write Key.vi"("section"=w339, "value"=w330, "key"="FrameRate", "refnum"=w341) -> ("refnum out"=w340:T13)  [unwired: 1 in, 6 out]
            n213 = property on="Camera Settings" class="Clust (strict)"("Visible"=w342) -> ()  [unwired: 2 in, 2 out]
            n214 = local write "DB Camera Config"(w342) -> ()
            n215 = call-poly <vilib>:"Write Key.vi"("section"=w339, "value"=w329, "key"="Compression", "refnum"=w340) -> ("refnum out"=w326:T13)  [unwired: 1 in, 6 out]
            n216 = call <vilib>:"Close Config Data.vi"("refnum"=w326) -> ("file path"=w327:path)  [unwired: 2 in, 8 out]
            n217 = call <vilib>:"Open Config Data.vi"("configuration file path"=w327) -> ("refnum"=w325:T13)  [unwired: 8 in, 2 out]
          }
          frame True {
            n218 = property on="Camera Settings" class="Clust (strict)"("Visible"=TRUE) -> ()  [unwired: 2 in, 2 out]
          }
        }
      }
      event "Camera Settings": Value Change {
        n219 = event-data() -> ("NewVal"=w356:T2)  [unwired: 1 in]
        n220 = Index Array(array=w352) -> (element=w351:cluster{string[]})  [unwired: 1 in]
        n221 = Unbundle(w356) -> ("Frame Rate"=w347:i32, "Compression"=w346:i32, "Size"=w349:u16)
        n222 = Unbundle(w351) -> (w350:string[])
        n223 = Index Array(array=w350, index=w349) -> (element=w348:string)
        n224 = Format Into String(format string="%s   %dfps   %d%%", w348, w347, w346) -> (resulting string=w353:string)  [unwired: 2 in, 1 out]
        n225 = Build Array(w353) -> (w354:string[])
        n226 = property on="DB Camera Config" class="Bool (strict)"("Strings [4]"=w354) -> ()  [unwired: 2 in, 2 out]
      }
      event "Motor.Enable": Value Change {
        n227 = event-data() -> ("NewVal"=w362:bool)  [unwired: 1 in]
        n228 = Unbundle("Motor") -> ("Value"=w361:dbl)  [unwired: 1 out]
        n229 = Select(t=w361, s=w362, f=0.0) -> (s? t:f=w359:dbl)
        n230 = call <vilib>:"NT Write Number.vi"("Numeric"=w359, "Name"=w358) -> ()  [unwired: 9 in, 1 out]
      }
      event "Test Slider": Value Change {
        n231 = event-data() -> ("NewVal"=w365:dbl)  [unwired: 1 in]
        n232 = call <vilib>:"NT Write Number.vi"("Numeric"=w365, "Name"=w366) -> ()  [unwired: 9 in, 1 out]
      }
      event "On/Off": Value Change {
        n233 = event-data() -> ("NewVal"=w370:bool)  [unwired: 1 in]
        n234 = Boolean To (0,1)(Boolean=w370) -> (0, 1=w369:i16)
        n235 = call <vilib>:"NT Write Number.vi"("Numeric"=w369, "Name"=w368) -> ()  [unwired: 9 in, 1 out]
      }
      event "Rev/Fwd": Value Change {
        n236 = event-data() -> ("NewVal.Forward"=w378:bool, "NewVal.Reverse"=w377:bool)  [unwired: 1 in]
        n237 = Boolean To (0,1)(Boolean=w378) -> (0, 1=w374:i16)
        n238 = Boolean To (0,1)(Boolean=w377) -> (0, 1=w376:i16)
        n239 = Negate(x=w376) -> (-x=w375:i16)
        n240 = Add(x=w374, y=w375) -> (x+y=w373:i16)
        n241 = call <vilib>:"NT Write Number.vi"("Numeric"=w373, "Name"=w372) -> ()  [unwired: 9 in, 1 out]
      }
      event "Test Ring": Value Change {
        n242 = event-data() -> ("NewVal"=w382:u16)  [unwired: 1 in]
        n243 = property on="Test Ring" class="Ring (strict)"() -> ("Strings []"=w383:string[])  [unwired: 2 in, 2 out]
        n244 = Index Array(array=w383, index=w382) -> (element=w381:string)
        n245 = call <vilib>:"NT Write String.vi"("String"=w381, "Name"=w380) -> ()  [unwired: 9 in, 1 out]
      }
      event "Rec Mode": Value Change {
        # "Update globals for recording mode and path to read log from.\nClear when logging and let NetworkTables set path for vision to\nuse."
        n246 = event-data() -> ("NewVal"=w393:enum32{"Stop", "Record", "Playback"})  [unwired: 1 in]
        n247 = case shown="\"Stop\", \"Record\"" w393 {
          tunnel: w392 -> [_ w395 w403]
          tunnel: [_ _ w402] -> w389
          tunnel: [_ _ w401] -> _
          tunnel: w387 -> [_ _ w399]
          tunnel: cluster{i32, i32} {-250, 170} -> [_ _ w398]
          tunnel: [_ _ T15 {"Image Size"=TRUE, "Image Type"=TRUE, "Pixel Value"=TRUE, "ROI Information"=TRUE, "Zoom Factor"=FALSE} ("Image Information Shown:All Elements")] -> w385
          tunnel: [_ _ TRUE ("Zoom Factor")] -> w384
          frame Default {
          }
          frame "Stop", "Record" {
            # "Place Window too"
            n248 = invoke class="VI" method="FP.Close"(reference=w395) -> (reference out=w394:refnum<vi>)  [unwired: 2 in, 2 out]
            n249 = invoke class="VI" method="Abort VI"(reference=w394) -> ()  [unwired: 2 in, 3 out]
          }
          frame "Playback" {
            n250 = call "Open Playback Panel.vi"("Offset"=w398, "DB VI Ref"=w399, "Playback in"=w403) -> ("Playback out"=w400:refnum<vi>)  [unwired: 8 in]
            n251 = register-events(w400) -> (reference out=w402:refnum<event-registration>, error out=w401:errorcluster)  [unwired: 2 in]
          }
        }
        n252 = global write "WPI_DashboardLogging Global.vi" "Recording"(w393) -> ()
        n253 = global write "WPI_DashboardLogging Global.vi" "Logging Filename"(path "") -> ()
        n254 = property on="Camera Image" class="ImageControl"("Image Information Shown"=w385, "Image Information Visible"=w384) -> ()  [unwired: 2 in, 2 out]
        n255 = call <vilib>:"WPI_DashboardNT Log FieldName Cache.vi"("Operation"=enum16{"Lookup/Add", "Index", "Clear"}."Clear") -> ()  [unwired: 8 in, 3 out]
      }
      event Panel Close {
        w404 = enum32{"Stop", "Record", "Playback"}."Stop" ("Rec Mode")
        n256 = event-data() -> ()  [unwired: 1 in, 4 out]
        n257 = local write "Rec Mode"(w404) -> ()
        n258 = global write "WPI_DashboardLogging Global.vi" "Recording"(w404) -> ()
      }
      event Panel Close {
        # "Abort playback window and ourself"
        n259 = event-data() -> ()  [unwired: 1 in, 4 out]
        n260 = invoke class="VI" method="FP.Close"(reference=w409) -> (reference out=w408:refnum<vi>)  [unwired: 2 in, 2 out]
        n261 = invoke class="VI" method="Abort VI"(reference=w408) -> (error out=w407:errorcluster)  [unwired: 2 in, 2 out]
        n262 = invoke class="VI" method="Abort VI"(error in=w407) -> ()  [unwired: 2 in, 3 out]
      }
    }
  }
  n263 = property on="On/Off" class="Bool (strict)"("Visible"=w25) -> ()  [unwired: 2 in, 2 out]
  n264 = property on="Motor" class="Clust (strict)"("Visible"=w25) -> ()  [unwired: 2 in, 2 out]
  n265 = property on="Progress" class="Clust (strict)"("Visible"=w25) -> ()  [unwired: 2 in, 2 out]
  n266 = property on="Test Ring" class="Ring (strict)"("Visible"=w25) -> ()  [unwired: 2 in, 2 out]
  n267 = property on="Rev/Fwd" class="Clust (strict)"("Visible"=w25) -> ()  [unwired: 2 in, 2 out]
  n268 = property on="Camera Settings" class="Clust (strict)"("Visible"=w25) -> ()  [unwired: 2 in, 2 out]
  n269 = local write "DB Camera Config"(w25) -> ()
  n270 = global write "WPI_DashboardLogging Global.vi" "Recording"(w8) -> ()
  n271 = local write "Rec Mode"(w8) -> ()
